vi "Get Freq-Time Spectral Map (DBL).vi"(7 "dB On (T)":bool=TRUE, 8 "error in (no error)":errorcluster, 10 "sampling frequency [Hz]":dbl=1.0 format="%.2f", 11 "RefNum in":T1) -> (0 "error out":errorcluster, 1 "quantization info":cluster{"offset":dbl, "multiplier":dbl} {"multiplier" format="%.2f"; "offset" format="%.2f"}, 2 "spectral map":dbl[][](array[numeric]) format="%.2f", 3 "RefNum out":T1, 4 "frequency scale":cluster{"offset":dbl, "multiplier":dbl} {"multiplier" format="%.2f"; "offset" format="%.2f"}, 5 "time scale":cluster{"offset":dbl, "multiplier":dbl} {"multiplier" format="%.2f"; "offset" format="%.2f"})   [LabVIEW 2017, in "SoundVib_Gabor.lvlib"]
doc: "Generates a frequency-time spectral map of the data block referenced by <B>RefNum in</B>. You can use this polymorphic VI to return <B>spectral map</B> as a 2D array of double-precision, floating-point numbers or a 2D array of 8-bit unsigned integers. You must manually select the polymorphic instance to use. Use the DBL instance to obtain more accurate data. Use the U8 instance to reduce memory usage when the VI displays data."
uses:
  <vilib>/addons/Sound and Vibration/Order Analysis/Gabor Order Tracking/SoundVib_Gabor.lvlib
  <vilib>/addons/Sound and Vibration/Order Analysis/Ref Gabor Order Tracking/GT RefNum.ctl
  <resource>/sndvib.dll
panel:
  # "Get Freq-Time Spectral Map (DBL)"
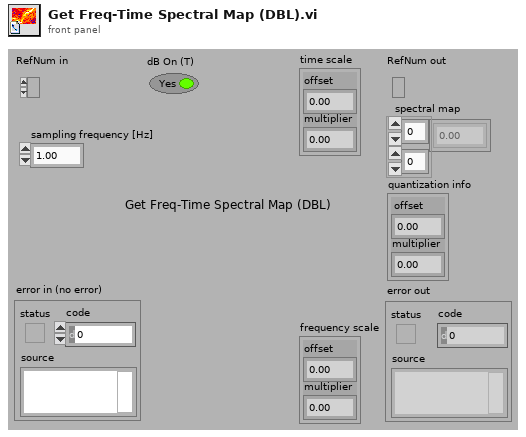
[diagram p1: front panel]
types:
  T1 = typedef "SoundVib_Gabor.lvlib/GT RefNum.ctl" = refnum<k1>
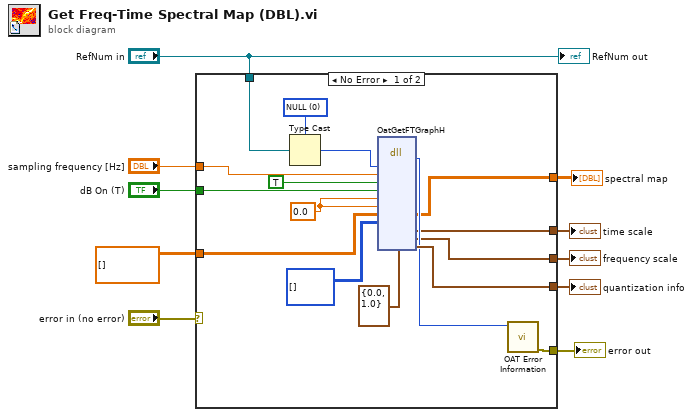
[diagram p0: block diagram]
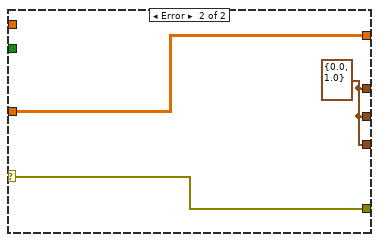
[diagram p2: hidden frame]
diagram:
  n1 = case shown="No Error" "error in (no error)" {
    selector: "error in (no error)" -> [_ w29]
    tunnel: [w26 w29] -> w10
    tunnel: "RefNum in" -> [w24 _]
    tunnel: "dB On (T)" -> [w21 _]
    tunnel: [w12 w28] -> w7
    tunnel: dbl[][] [] ("DBLGraph") -> [w20 w28]
    tunnel: [w15 w27] -> w6
    tunnel: [w14 w27] -> w5
    tunnel: [w17 w27] -> w4
    tunnel: "sampling frequency [Hz]" -> [w13 _]
    frame No Error {
      w18 = cluster{"Z Min":dbl, "Z Step":dbl} {"Z Min"=0.0, "Z Step"=1.0}
      w11 = 0.0
      w25 = u32 0 items=["NULL"]
      n2 = Type Cast(type=w25, x=w24) -> (*(type *) &x=w23:u32)
      n3 = dll-call lib="C:/Program Files (x86)/National Instruments/LabVIEW 2017/resource/sndvib.*" fn="OatGetFTGraphH"("Ref In"=w23, "Fs"=w13, "bGetDBL"=TRUE, "bLogZ"=w21, "UpperCutRatio"=w11, "LowerCutRatio"=w11, "DBLGraph"=w20, "U8Graph"=u8[][] [] ("Graph"), "XScale"=w18, "YScale"=w18, "ZScale"=w18) -> ("return type"=w16:i32, "DBLGraph"=w12:dbl[][], "XScale"=w15:cluster{"Z Min":dbl, "Z Step":dbl}, "YScale"=w14:cluster{"Z Min":dbl, "Z Step":dbl}, "ZScale"=w17:cluster{"Z Min":dbl, "Z Step":dbl})  [unwired: 10 in, 2 out]
      n4 = call <vilib>:"OAT Error Information.vi"("error code"=w16) -> ("error out"=w26:errorcluster)  [unwired: 6 in]
    }
    frame Error {
      w27 = cluster{"Z Min":dbl, "Z Step":dbl} {"Z Min"=0.0, "Z Step"=1.0}
    }
  }
  "error out" <- w10
  "spectral map" <- w7
  "quantization info" <- w4
  "frequency scale" <- w5
  "time scale" <- w6
  "RefNum out" <- "RefNum in"
